vi "TestExec.Result, Overwrite Test Result State.vi"(7 "Module Q Name":string, 8 "error in":errorcluster, 10 "ResultState":T1={"State"=enum."Passing", "Code"=0, "Description"=""}, 11 "Q In":refnum<queue>) -> (0 "error out":errorcluster)   [LabVIEW 2018]
uses:
  <vilib>/KATE/Queues/Q.Element.ctl
  <vilib>/KATE/SeqMgr/SeqMgr.Result Info.ctl
  <vilib>/KATE/SeqMgr/SeqMgr.Result State Enum.ctl
  <vilib>/KATE/Queues/Queue Utils.lvlib
  <vilib>/KATE/SeqMgr/SeqMgr.lvlib
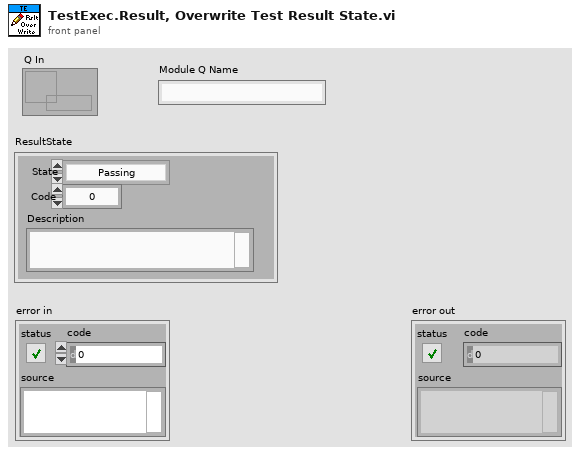
[diagram p1: front panel]
types:
  T1 = typedef "KATE_Lib.lvlib/SeqMgr.lvlib/SeqMgr.Result Info.ctl" = cluster{"State":T2, "Code":i32, "Description":string}
  T2 = typedef "KATE_Lib.lvlib/SeqMgr.lvlib/SeqMgr.Result State Enum.ctl" = enum16{"None", "Passing", "Failing", "PASS", "FAIL", "ABORT", "ERROR"}
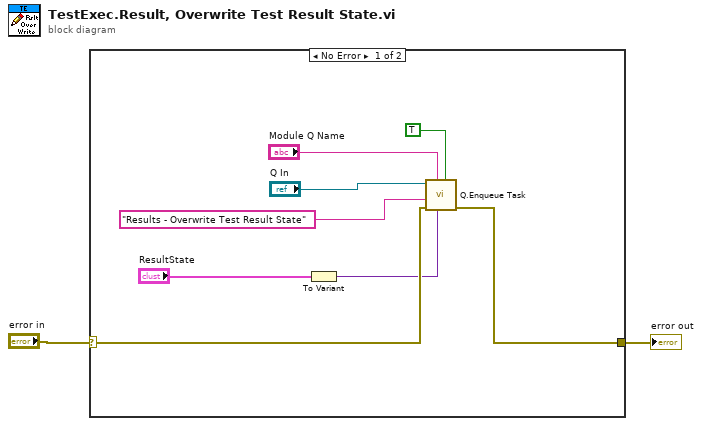
[diagram p0: block diagram]
diagram:
  n1 = case shown="No Error" "error in" {
    selector: "error in" -> [w7 w11]
    tunnel: [w8 w11] -> w1
    frame No Error {
      n2 = To Variant(anything="ResultState") -> (Variant=w6:variant)
      n3 = call <vilib>:"Q.Enqueue Task.vi"("Top of Q"=TRUE, "Data1"=w6, "Q Name"="Module Q Name", "Error In"=w7, "Task Name"="Results - Overwrite Test Result State" ("Cmd"), "Q In"="Q In") -> ("error out"=w8:errorcluster)  [unwired: 4 in, 1 out]
    }
    frame Error {
    }
  }
  "error out" <- w1
